vi "Pre Launch Init.vi"(11 "State Actor in":refnum<class "State Actor.lvclass">) -> (0 "error out":errorcluster, 3 "State Actor out":refnum<class "State Actor.lvclass">)   [LabVIEW 2024, in "State Actor.lvlib" / "State Actor.lvclass"]
doc: "<p>(<strong>Filename</strong>: <span class=\"dnl\">Actor Framework.lvlib:Actor.lvclass:Pre Launch Init.vi</span>)</p>\n<p>Defines behavior that occurs after the <a href=\"nihelplauncher://docs/csh?context=lvcore_lvcomm_af_launch_nested_actor\">Launch Nested Actor</a> method is invoked but before the actor's Actor Core method begins running.</p>\n<p>By default, this method does nothing. A descendant class may override it to define behavior.</p>"
uses:
  State Actor.lvclass
  State Transition Event.ctl
  State Actor.lvclass/State Actor.ctl
  <vilib>/ActorFramework/Actor/Actor.lvclass
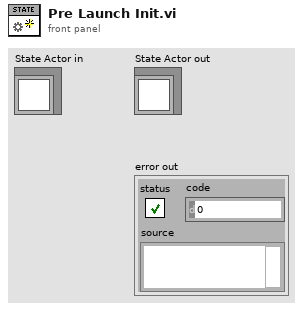
[diagram p1: front panel]
types:
  T1 = typedef "State Actor.lvlib/State Actor.lvclass/State Transition Event.ctl" = cluster{"Timestamp":timestamp, "State":string}
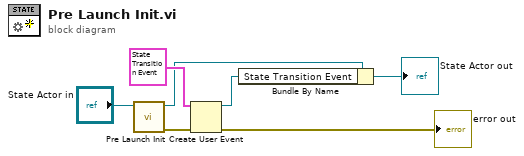
[diagram p0: block diagram]
diagram:
  n1 = call-parent "Pre Launch Init.vi"("Actor in"="State Actor in") -> ("error out"=w3:errorcluster, "Actor out"=w5:refnum<class "State Actor.lvclass">)  [unwired: 9 in]
  n2 = Create User Event(user event datatype=T1 {"Timestamp"=timestamp(0 s since 1904-01-01), "State"=""} ("State Transition Event"), error in=w3) -> (user event=w4:refnum<user-event>, error out=→"error out":errorcluster)
  n3 = Bundle By Name(cluster=w5, "State Transition Event"=w4) -> (→"State Actor out":refnum<class "State Actor.lvclass">)
